vi "Periodic Tasks.vi"(8 "error in":errorcluster) -> ()   [LabVIEW 2014]
doc: "This VI runs in parallel to other tasks. It can contain as many user-defined periodic loops as you need. These can carry out PID or other sorts of timed response."
uses:
  <vilib>/Rock Robotics/WPI/DriverStation/WPI_DriverStationRobotMode2.ctl
  <vilib>/Rock Robotics/WPI/Joystick/WPI_JoystickGetSetRefNum.vi
  <vilib>/Rock Robotics/WPI/RobotDrive/WPI_RobotDriveGetSetRefNum.vi
  <vilib>/Rock Robotics/Network Tables/SD Read Number.vi
  Robot Global Data.vi
  <vilib>/Rock Robotics/Network Tables/SD Write Number.vi
  <vilib>/addons/control/pid/pid.llb/PID (DBL).vi
  <vilib>/Rock Robotics/WPI/Solenoid/Deprecated/WPI_SolenoidSetBool.vi
  <vilib>/Rock Robotics/WPI/RobotDrive/WPI_RobotDriveMecanumDrive_Cartesian.vi
  <vilib>/Rock Robotics/Network Tables/SD Write Numeric Array.vi
  <vilib>/Rock Robotics/Network Tables/SD Write Boolean Array.vi
  <vilib>/Rock Robotics/Network Tables/SD Write Boolean.vi
  <vilib>/addons/control/pid/NI_PID_pid.lvlib
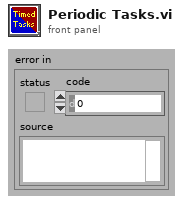
[diagram p1: front panel]
types:
  T1 = typedef "WPI_JoystickDevRef.ctl" = cluster{"Device":T2}
  T2 = typedef "WPI_JoystickDeviceEnum.ctl" = enum16{"USB 0", "USB 1", "USB 2", "USB 3", "USB 4", "USB 5"}
  T3 = typedef "WPI_RobotDriveDevRef.ctl" = cluster{"DevStatus":errorcluster, "Motors[]":T4[], "Square Inputs":bool, "Max Output":dbl}
  T4 = typedef "WPI_MotorControlDeviceRef.ctl" = cluster{"DeviceStatus":errorcluster, "Type":T5, "PWM":cluster{"Controller":T6, "PWM Channel":T7, "DeadBand":T8}, "CAN":cluster{"Device Number":u8, "Control Mode":T9, "Semaphore":T10, "Max Vout":dbl, "TalonSRX Control Mode":T11}, "Invert":bool, "TransformRef":T12, "InvTransformRef":T12}
  T5 = typedef "WPI_MotorControlType.ctl" = enum16{"PWM", "CAN", "CANTalonSRX"}
  T6 = typedef "FPGA_TypedefDigitalModule.ctl" = enum16{"Controller 1"}
  T7 = typedef "FPGA_DIOPWMChannel.ctl" = enum8{"PWM 0", "PWM 1", "PWM 2", "PWM 3", "PWM 4", "PWM 5", "PWM 6", "PWM 7", "PWM 8", "PWM 9", "PWM MXP 0", "PWM MXP 1", "PWM MXP 2", "PWM MXP 3", "PWM MXP 4", "PWM MXP 5", "PWM MXP 6", "PWM MXP 7", "PWM MXP 8", "PWM MXP 9", "Invalid"}
  T8 = typedef "WPI_PWMDeadband.ctl" = cluster{"Name":string, "maxPositivePwm":i32, "minPositivePwm":i32, "centerPwm":i32, "maxNegativePwm":i32, "minNegativePwm":i32, "angularRange":u16}
  T9 = typedef "WPI_CANJaguar_ControlMode.ctl" = enum8{"Percent VBus", "Current", "Speed", "Position", "Voltage"}
  T10 = typedef "Semaphore RefNum" = refnum<k1>
  T11 = typedef "WPI_CANTalonSRX_APIControlMode.ctl" = enum8{"Percent VBus", "Speed", "Position", "Slave", "Unchanged / Invalid"}
  T12 = typedef "WPI_PWMTransform_ConPane.ctl" = refnum<vi>
  T13 = typedef "WPI_EncoderDevRef.ctl" = cluster{"DevStatus":errorcluster, "EncoderIndex":T14, "CounterIndex":T15, "DistancePerCount":dbl, "Decoding Type":T16}
  T14 = typedef "FPGA_EncoderIdx.ctl" = enum8{"Enc 0", "Enc 1", "Enc 2", "Enc 3", "Enc 4", "Enc 5", "Enc 6", "Enc 7", "Invalid"}
  T15 = typedef "FPGA_CounterCtrSystemIndex.ctl" = enum8{"Ctr 0", "Ctr 1", "Ctr 2", "Ctr 3", "Ctr 4", "Ctr 5", "Ctr 6", "Ctr 7", "Invalid"}
  T16 = typedef "WPI_EncoderType.ctl" = enum16{"1x", "2x", "4x"}
  T17 = typedef "WPI_GyroDevRef.ctl" = cluster{"DevStatus":errorcluster, "Analog Module":T18, "Analog Channel":T19, "Offset":dbl, "Gain (VoltsPerDegree/Second)":dbl}
  T18 = typedef "FPGA_TypedefAnalogModule.ctl" = enum16{"Controller 1"}
  T19 = typedef "FPGA_AIChannel.ctl" = enum8{"AI 0", "AI 1", "AI 2", "AI 3", "AI MXP 0", "AI MXP 1", "AI MXP 2", "AI MXP 3", "Invalid"}
  T20 = typedef "WPI_SwitchDevRef.ctl" = cluster{"DevStatus":errorcluster, "DIO Channel":T21, "Controller":T6, "CntIndex":T15, "Normally Closed":bool}
  T21 = typedef "FPGA_DIOChannel.ctl" = enum8{"DIO 0", "DIO 1", "DIO 2", "DIO 3", "DIO 4", "DIO 5", "DIO 6", "DIO 7", "DIO 8", "DIO 9", "DIO MXP 0", "DIO MXP 1", "DIO MXP 2", "DIO MXP 3", "DIO MXP 4", "DIO MXP 5", "DIO MXP 6", "DIO MXP 7", "DIO MXP 8", "DIO MXP 9", "DIO MXP 10", "DIO MXP 11", "DIO MXP 12", "DIO MXP 13", "DIO MXP 14", "DIO MXP 15", "Invalid"}
  T22 = typedef "WPI_SolenoidDevRef.ctl" = cluster{"DevStatus":errorcluster, "Pneumatics Control Module":u8, "Forward Solenoid Channel":T23, "Reverse Solenoid Channel":T23}
  T23 = typedef "WPI_SolenoidChannel.ctl" = enum8{"Solenoid 0", "Solenoid 1", "Solenoid 2", "Solenoid 3", "Solenoid 4", "Solenoid 5", "Solenoid 6", "Solenoid 7", "Invalid"}
  T24 = cluster{"JoystickDevRef":T1, "RobotDriveDevRef":T3}
  T25 = cluster{"Buttons[0]":bool, "Buttons[1]":bool, "Buttons[2]":bool, "Buttons[3]":bool, "Buttons[4]":bool, "Buttons[5]":bool, "Buttons[6]":bool, "Buttons[7]":bool, "Buttons[8]":bool}
  T26 = typedef "WPI_DriverStationRobotMode2.ctl" = enum16{"Autonomous Disabled", "Autonomous Enabled", "Teleop Disabled", "Teleop Enabled", "Disconnected", "Finish", "Test Disabled", "Test Enabled", "Emergency Stopped"}
  T27 = cluster{"proportional gain (Kc)":dbl, "integral time (Ti, min)":dbl, "derivative time (Td, min)":dbl}
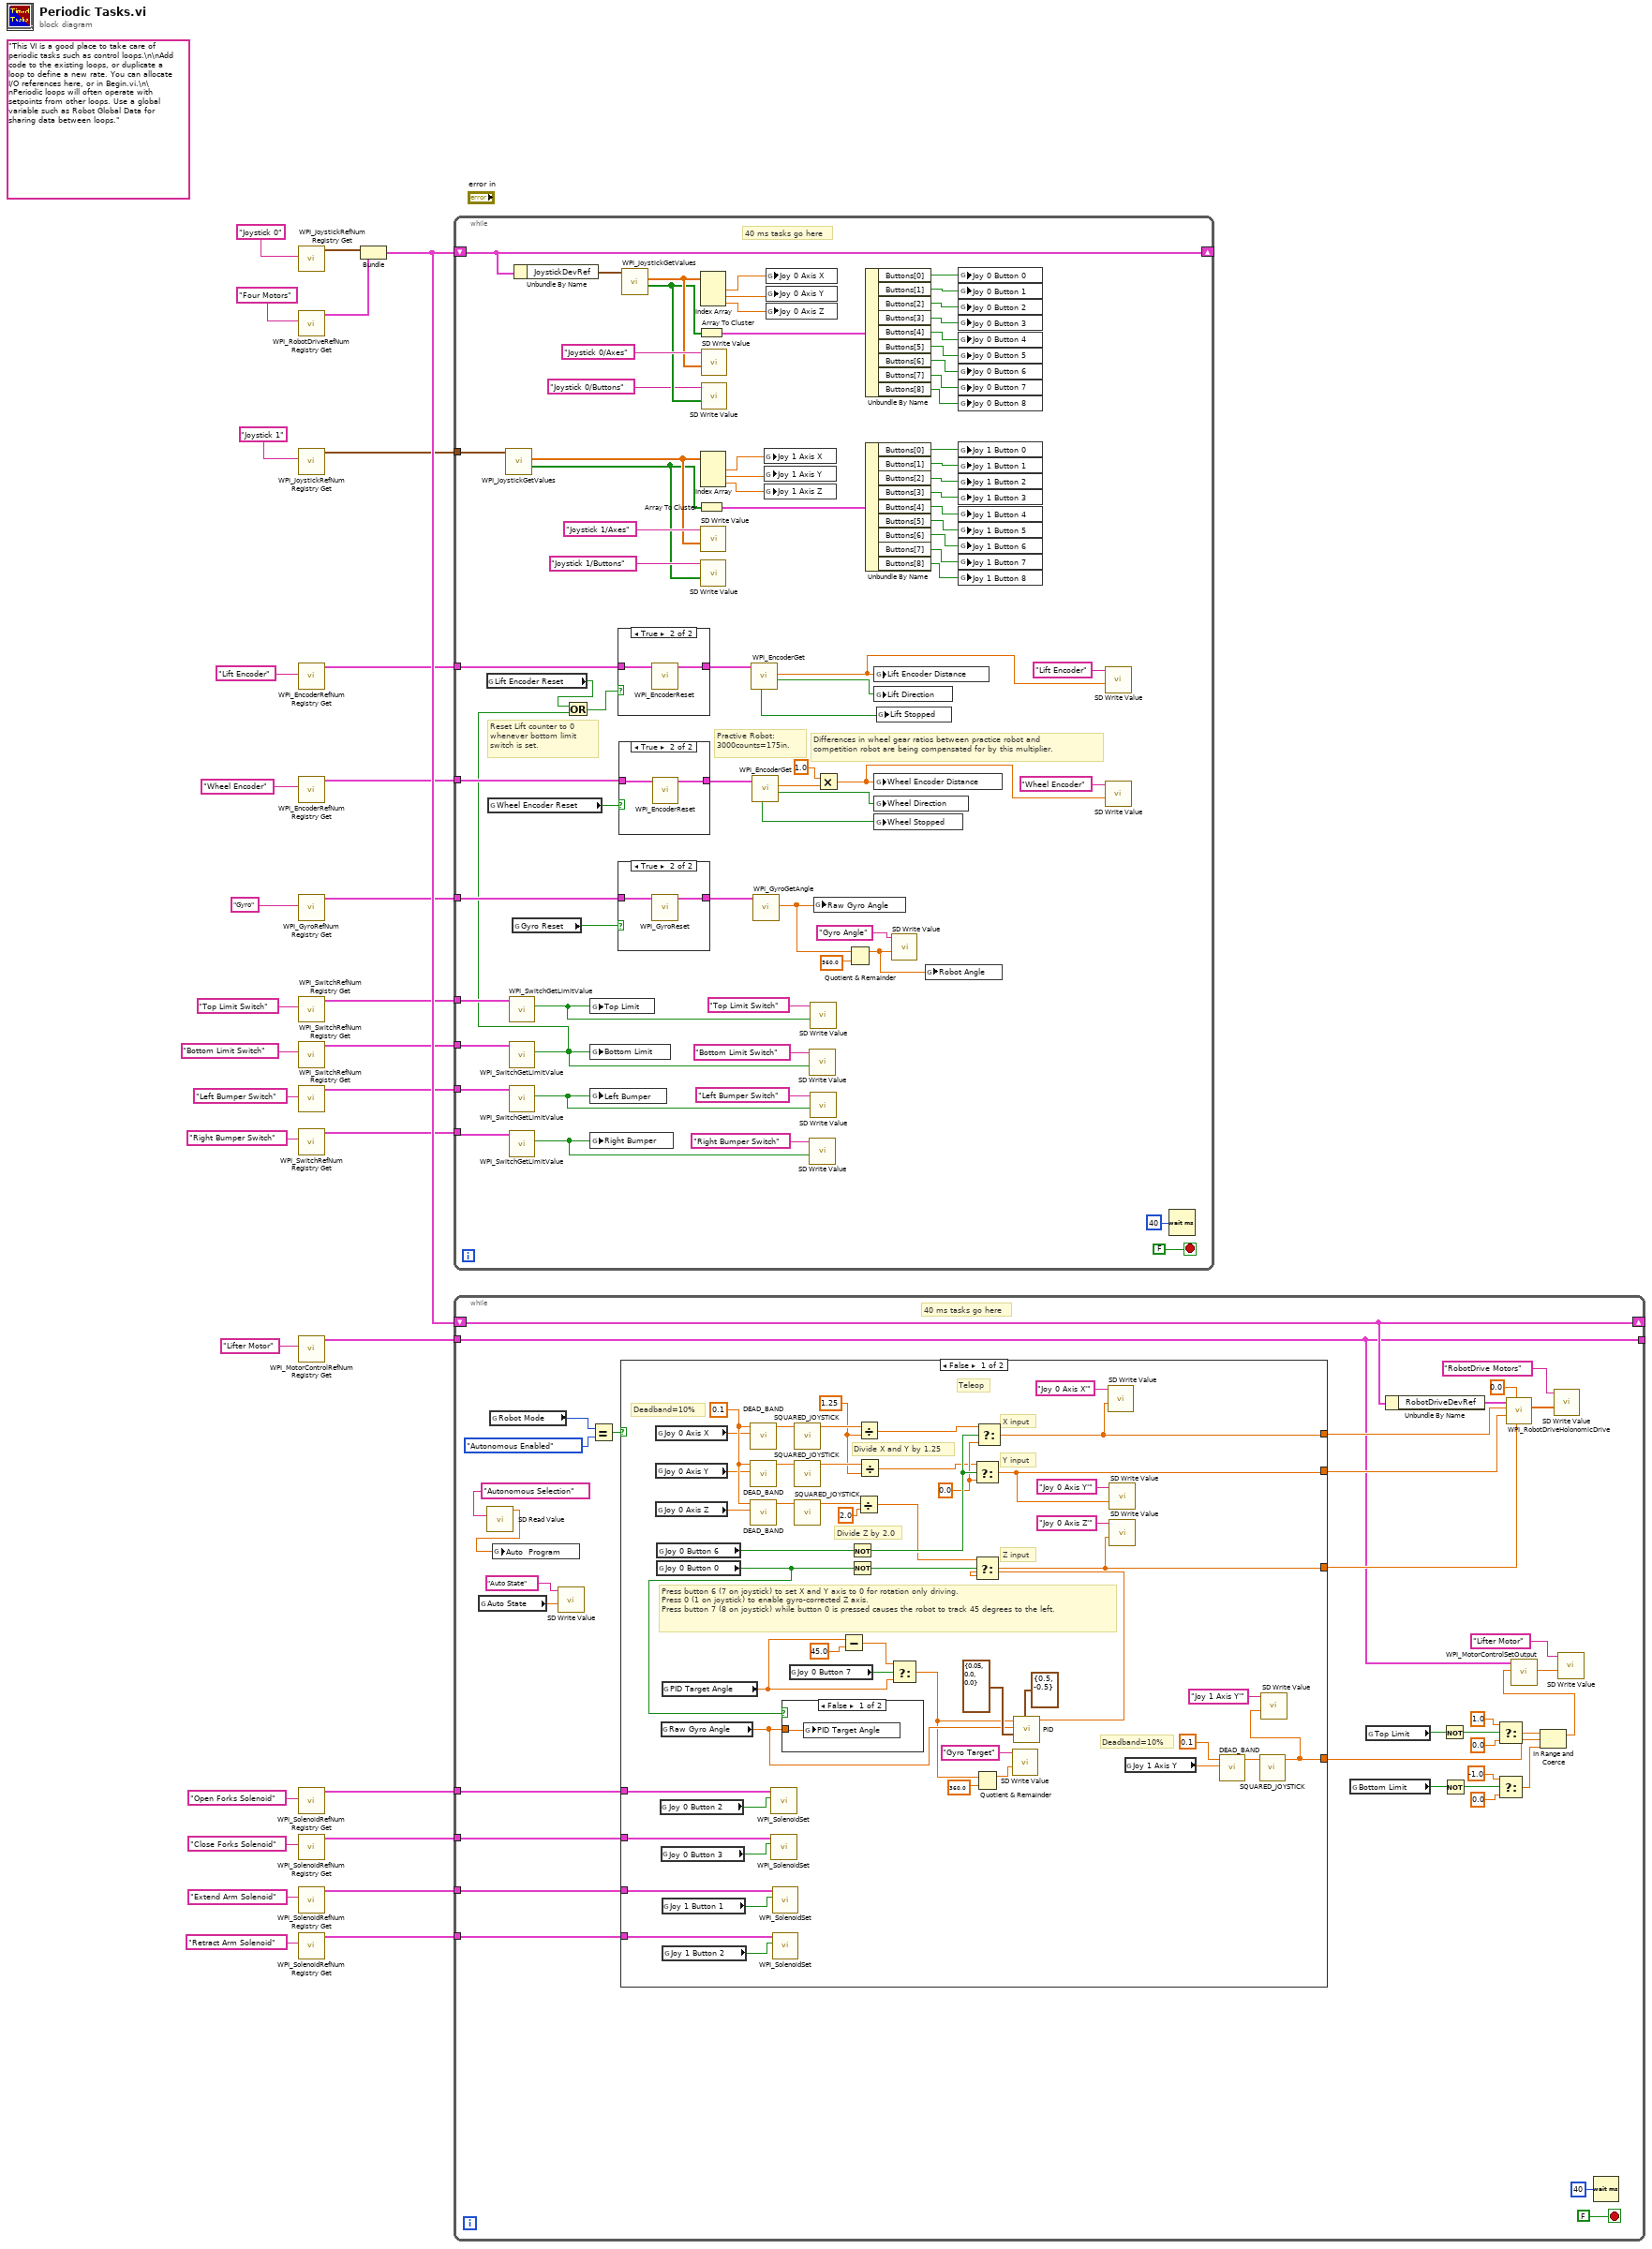
[diagram p0: block diagram]
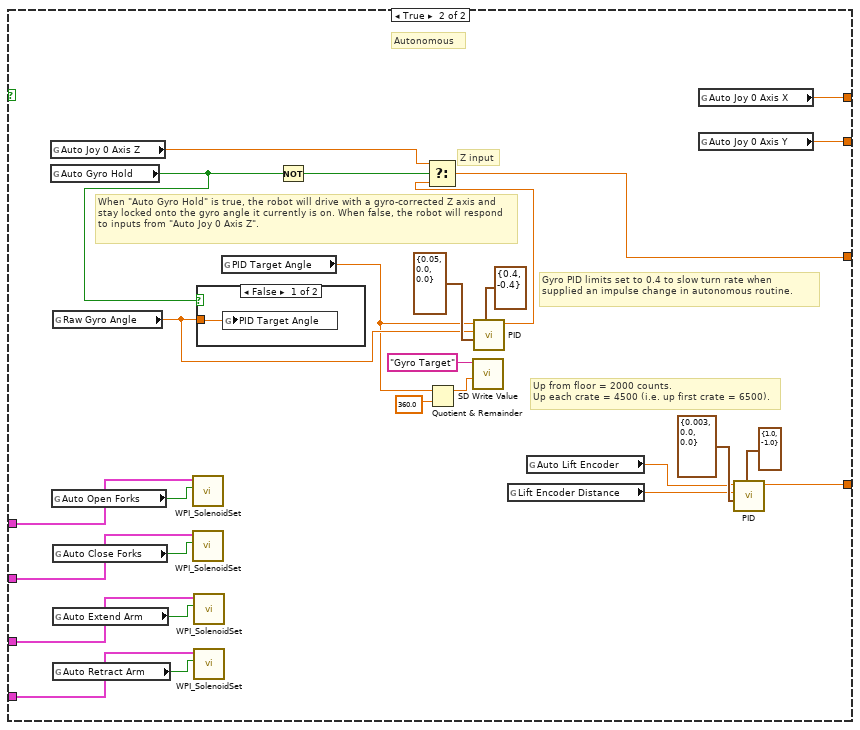
[diagram p3: hidden frame]
diagram:
  (unwired) "This VI is a good place to take care of periodic tasks such as control loops.\n\nAdd code to the existing loops, or duplicate a loop to define a new rate. You can allocate I/O references here, or in Begin.vi.\n\nPeriodic loops will often operate with setpoints from other loops. Use a global variable such as Robot Global Data for sharing data between loops."
  n1 = call <vilib>:"WPI_JoystickRefNum Registry Get.vi"("refnum name"="Joystick 0") -> ("JoystickDevRef"=w29:T1)  [unwired: 1 in, 9 out]
  n2 = call <vilib>:"WPI_RobotDriveRefNum Registry Get.vi"("refnum name"="Four Motors") -> ("RobotDriveDevRef"=w28:T3)  [unwired: 1 in, 9 out]
  n3 = call <vilib>:"WPI_JoystickRefNum Registry Get.vi"("refnum name"="Joystick 1") -> ("JoystickDevRef"=w25:T1)  [unwired: 1 in, 9 out]
  n4 = call <vilib>:"WPI_EncoderRefNum Registry Get.vi"("refnum name"="Lift Encoder") -> ("EncoderDevRef"=w21:T13)  [unwired: 9 in, 1 out]
  n5 = call <vilib>:"WPI_EncoderRefNum Registry Get.vi"("refnum name"="Wheel Encoder") -> ("EncoderDevRef"=w19:T13)  [unwired: 9 in, 1 out]
  n6 = call <vilib>:"WPI_GyroRefNum Registry Get.vi"("refnum name"="Gyro") -> ("GyroDevRef"=w23:T17)  [unwired: 9 in, 1 out]
  n7 = call <vilib>:"WPI_SwitchRefNum Registry Get.vi"("refnum name"="Top Limit Switch") -> ("SwitchDevRef"=w17:T20)  [unwired: 9 in, 1 out]
  n8 = call <vilib>:"WPI_SwitchRefNum Registry Get.vi"("refnum name"="Bottom Limit Switch") -> ("SwitchDevRef"=w16:T20)  [unwired: 9 in, 1 out]
  n9 = call <vilib>:"WPI_SwitchRefNum Registry Get.vi"("refnum name"="Left Bumper Switch") -> ("SwitchDevRef"=w2:T20)  [unwired: 9 in, 1 out]
  n10 = call <vilib>:"WPI_SwitchRefNum Registry Get.vi"("refnum name"="Right Bumper Switch") -> ("SwitchDevRef"=w1:T20)  [unwired: 9 in, 1 out]
  n11 = call <vilib>:"WPI_MotorControlRefNum Registry Get.vi"("refnum name"="Lifter Motor") -> ("MotorControlDevRef"=w5:T4)  [unwired: 9 in, 1 out]
  n12 = call <vilib>:"WPI_SolenoidRefNum Registry Get.vi"("refnum name"="Open Forks Solenoid") -> ("SolenoidDevRef"=w12:T22)  [unwired: 9 in, 1 out]
  n13 = call <vilib>:"WPI_SolenoidRefNum Registry Get.vi"("refnum name"="Close Forks Solenoid") -> ("SolenoidDevRef"=w11:T22)  [unwired: 9 in, 1 out]
  n14 = call <vilib>:"WPI_SolenoidRefNum Registry Get.vi"("refnum name"="Extend Arm Solenoid") -> ("SolenoidDevRef"=w8:T22)  [unwired: 9 in, 1 out]
  n15 = call <vilib>:"WPI_SolenoidRefNum Registry Get.vi"("refnum name"="Retract Arm Solenoid") -> ("SolenoidDevRef"=w7:T22)  [unwired: 9 in, 1 out]
  n16 = Bundle("JoystickDevRef"=w29, "RobotDriveDevRef"=w28) -> (w27:T24)  [unwired: 1 out]
  n17 = while {
    shift-right: [w104] -> _
    shift-left: w27 -> [w104]
    tunnel: w25 -> [w89]
    tunnel: w23 -> [w75]
    tunnel: w21 -> [w72]
    tunnel: w19 -> [w69]
    tunnel: w17 -> [w55]
    tunnel: w16 -> [w54]
    tunnel: w2 -> [w40]
    tunnel: w1 -> [w39]
    stop <- FALSE stop-if-true
    # "Practive Robot:\n3000counts=175in."
    # "Differences in wheel gear ratios between practice robot and competition robot are being compensated for by this multiplier."
    # "Reset Lift counter to 0 whenever bottom limit switch is set."
    # "40 ms tasks go here"
    n18 = global read "Robot Global Data.vi" "Lift Encoder Reset"() -> (w36:bool)
    n19 = global read "Robot Global Data.vi" "Wheel Encoder Reset"() -> (w70:bool)
    n20 = call <vilib>:"WPI_JoystickGetValues.vi"("JoystickDevRef"=w89) -> ("Buttons"=w60:bool[], "Axes"=w61:dbl[])  [unwired: 6 in, 3 out]
    n21 = call <vilib>:"WPI_SwitchGetLimitValue.vi"("SwitchDevRef"=w55) -> ("Switch Pressed"=w51:bool)  [unwired: 8 in, 2 out]
    n22 = call <vilib>:"WPI_SwitchGetLimitValue.vi"("SwitchDevRef"=w54) -> ("Switch Pressed"=w35:bool)  [unwired: 8 in, 2 out]
    n23 = call <vilib>:"WPI_SwitchGetLimitValue.vi"("SwitchDevRef"=w40) -> ("Switch Pressed"=w43:bool)  [unwired: 8 in, 2 out]
    n24 = call <vilib>:"WPI_SwitchGetLimitValue.vi"("SwitchDevRef"=w39) -> ("Switch Pressed"=w44:bool)  [unwired: 8 in, 2 out]
    n25 = global read "Robot Global Data.vi" "Gyro Reset"() -> (w73:bool)
    n26 = Unbundle By Name(w104) -> ("JoystickDevRef"=w103:T1)
    n27 = Or(x=w36, y=w35) -> (x .or. y?=w37:bool)
    n28 = global write "Robot Global Data.vi" "Top Limit"(w51) -> ()
    n29 = global write "Robot Global Data.vi" "Bottom Limit"(w35) -> ()
    n30 = global write "Robot Global Data.vi" "Left Bumper"(w43) -> ()
    n31 = global write "Robot Global Data.vi" "Right Bumper"(w44) -> ()
    n32 = case shown="True" w37 {
      tunnel: w72 -> [w110 w112]
      tunnel: [w110 w111] -> w71
      frame False {
      }
      frame True {
        n33 = call <vilib>:"WPI_EncoderReset.vi"("EncoderDevRef"=w112) -> ("EncoderDevRef"=w111:T13)  [unwired: 9 in, 1 out]
      }
    }
    n34 = case shown="True" w73 {
      tunnel: w75 -> [w113 w115]
      tunnel: [w113 w114] -> w74
      frame False {
      }
      frame True {
        n35 = call <vilib>:"WPI_GyroReset.vi"("GyroDevRef"=w115) -> ("GyroDevRef"=w114:T17)  [unwired: 9 in, 1 out]
      }
    }
    n36 = case shown="True" w70 {
      tunnel: w69 -> [w107 w108]
      tunnel: [w107 w109] -> w68
      frame False {
      }
      frame True {
        n37 = call <vilib>:"WPI_EncoderReset.vi"("EncoderDevRef"=w108) -> ("EncoderDevRef"=w109:T13)  [unwired: 9 in, 1 out]
      }
    }
    n38 = call <vilib>:"WPI_JoystickGetValues.vi"("JoystickDevRef"=w103) -> ("Buttons"=w65:bool[], "Axes"=w66:dbl[])  [unwired: 6 in, 3 out]
    n39 = Array To Cluster(array=w65) -> (cluster=w102:T25)
    n40 = Array To Cluster(array=w60) -> (cluster=w88:T25)
    n41 = Index Array(array=w66) -> (element #1=w92:dbl, element #2=w91:dbl, element #3=w90:dbl)  [unwired: 3 in]
    n42 = Index Array(array=w61) -> (element #1=w78:dbl, element #2=w77:dbl, element #3=w76:dbl)  [unwired: 3 in]
    n43 = call-poly <vilib>:"SD Write Value.vi"("Numeric Array"=w61, "Name"="Joystick 1/Axes") -> ()  [unwired: 8 in, 2 out]
    n44 = call-poly <vilib>:"SD Write Value.vi"("Boolean Array"=w60, "Name"="Joystick 1/Buttons") -> ()  [unwired: 8 in, 2 out]
    n45 = call-poly <vilib>:"SD Write Value.vi"("Numeric Array"=w66, "Name"="Joystick 0/Axes") -> ()  [unwired: 8 in, 2 out]
    n46 = call-poly <vilib>:"SD Write Value.vi"("Boolean Array"=w65, "Name"="Joystick 0/Buttons") -> ()  [unwired: 8 in, 2 out]
    n47 = call <vilib>:"WPI_EncoderGet.vi"("EncoderDevRef"=w71) -> ("Direction"=w50:bool, "Distance"=w38:dbl, "Stopped"=w49:bool)  [unwired: 5 in, 3 out]
    n48 = call <vilib>:"WPI_EncoderGet.vi"("EncoderDevRef"=w68) -> ("Direction"=w48:bool, "Distance"=w34:dbl, "Stopped"=w47:bool)  [unwired: 5 in, 3 out]
    n49 = call <vilib>:"WPI_GyroGetAngle.vi"("GyroDevRef"=w74) -> ("Angle"=w57:dbl)  [unwired: 7 in, 3 out]
    n50 = global write "Robot Global Data.vi" "Joy 1 Axis X"(w78) -> ()
    n51 = global write "Robot Global Data.vi" "Joy 1 Axis Y"(w77) -> ()
    n52 = global write "Robot Global Data.vi" "Joy 1 Axis Z"(w76) -> ()
    n53 = global write "Robot Global Data.vi" "Joy 0 Axis X"(w92) -> ()
    n54 = global write "Robot Global Data.vi" "Joy 0 Axis Y"(w91) -> ()
    n55 = global write "Robot Global Data.vi" "Joy 0 Axis Z"(w90) -> ()
    n56 = call-poly <vilib>:"SD Write Value.vi"("Boolean"=w35, "Name"="Bottom Limit Switch") -> ()  [unwired: 8 in, 2 out]
    n57 = call-poly <vilib>:"SD Write Value.vi"("Boolean"=w44, "Name"="Right Bumper Switch") -> ()  [unwired: 8 in, 2 out]
    n58 = call-poly <vilib>:"SD Write Value.vi"("Boolean"=w51, "Name"="Top Limit Switch") -> ()  [unwired: 8 in, 2 out]
    n59 = call-poly <vilib>:"SD Write Value.vi"("Boolean"=w43, "Name"="Left Bumper Switch") -> ()  [unwired: 8 in, 2 out]
    n60 = global write "Robot Global Data.vi" "Raw Gyro Angle"(w57) -> ()
    n61 = Multiply(x=1.0, y=w34) -> (x*y=w33:dbl)
    n62 = Quotient & Remainder(x=w57, y=360.0) -> (x-y*floor(x/y)=w56:dbl)  [unwired: 1 out]
    n63 = Unbundle By Name(w102) -> ("Buttons[0]"=w101:bool, "Buttons[1]"=w100:bool, "Buttons[2]"=w99:bool, "Buttons[3]"=w98:bool, "Buttons[4]"=w97:bool, "Buttons[5]"=w96:bool, "Buttons[6]"=w95:bool, "Buttons[7]"=w94:bool, "Buttons[8]"=w93:bool)
    n64 = Unbundle By Name(w88) -> ("Buttons[0]"=w87:bool, "Buttons[1]"=w86:bool, "Buttons[2]"=w85:bool, "Buttons[3]"=w84:bool, "Buttons[4]"=w83:bool, "Buttons[5]"=w82:bool, "Buttons[6]"=w81:bool, "Buttons[7]"=w80:bool, "Buttons[8]"=w79:bool)
    n65 = global write "Robot Global Data.vi" "Lift Encoder Distance"(w38) -> ()
    n66 = global write "Robot Global Data.vi" "Lift Direction"(w50) -> ()
    n67 = global write "Robot Global Data.vi" "Wheel Encoder Distance"(w33) -> ()
    n68 = global write "Robot Global Data.vi" "Wheel Direction"(w48) -> ()
    n69 = global write "Robot Global Data.vi" "Wheel Stopped"(w47) -> ()
    n70 = global write "Robot Global Data.vi" "Lift Stopped"(w49) -> ()
    n71 = call-poly <vilib>:"SD Write Value.vi"("Numeric"=w56, "Name"="Gyro Angle") -> ()  [unwired: 8 in, 2 out]
    n72 = global write "Robot Global Data.vi" "Robot Angle"(w56) -> ()
    n73 = global write "Robot Global Data.vi" "Joy 0 Button 0"(w101) -> ()
    n74 = global write "Robot Global Data.vi" "Joy 0 Button 1"(w100) -> ()
    n75 = global write "Robot Global Data.vi" "Joy 0 Button 2"(w99) -> ()
    n76 = global write "Robot Global Data.vi" "Joy 0 Button 3"(w98) -> ()
    n77 = global write "Robot Global Data.vi" "Joy 0 Button 4"(w97) -> ()
    n78 = global write "Robot Global Data.vi" "Joy 0 Button 5"(w96) -> ()
    n79 = global write "Robot Global Data.vi" "Joy 0 Button 6"(w95) -> ()
    n80 = global write "Robot Global Data.vi" "Joy 0 Button 7"(w94) -> ()
    n81 = global write "Robot Global Data.vi" "Joy 0 Button 8"(w93) -> ()
    n82 = global write "Robot Global Data.vi" "Joy 1 Button 0"(w87) -> ()
    n83 = global write "Robot Global Data.vi" "Joy 1 Button 1"(w86) -> ()
    n84 = global write "Robot Global Data.vi" "Joy 1 Button 2"(w85) -> ()
    n85 = global write "Robot Global Data.vi" "Joy 1 Button 3"(w84) -> ()
    n86 = global write "Robot Global Data.vi" "Joy 1 Button 4"(w83) -> ()
    n87 = global write "Robot Global Data.vi" "Joy 1 Button 5"(w82) -> ()
    n88 = global write "Robot Global Data.vi" "Joy 1 Button 6"(w81) -> ()
    n89 = global write "Robot Global Data.vi" "Joy 1 Button 7"(w80) -> ()
    n90 = global write "Robot Global Data.vi" "Joy 1 Button 8"(w79) -> ()
    n91 = call-poly <vilib>:"SD Write Value.vi"("Numeric"=w38, "Name"="Lift Encoder") -> ()  [unwired: 8 in, 2 out]
    n92 = call-poly <vilib>:"SD Write Value.vi"("Numeric"=w33, "Name"="Wheel Encoder") -> ()  [unwired: 8 in, 2 out]
    n93 = Wait (ms)(milliseconds to wait=u32 40) -> ()  [unwired: 1 out]
  }
  n94 = while {
    shift-right: [w146] -> _
    shift-left: w27 -> [w146]
    tunnel: w12 -> [w138]
    tunnel: w11 -> [w137]
    tunnel: w8 -> [w136]
    tunnel: w7 -> [w135]
    tunnel: [w134] -> _
    tunnel: w5 -> [w134]
    stop <- FALSE stop-if-true
    # "40 ms tasks go here"
    n95 = global read "Robot Global Data.vi" "Auto State"() -> (w117:dbl)
    n96 = call-poly <vilib>:"SD Read Value.vi"("Name"="Autonomous Selection") -> ("Numeric"=w118:dbl)  [unwired: 8 in, 2 out]
    n97 = global read "Robot Global Data.vi" "Robot Mode"() -> (w140:T26)
    n98 = global write "Robot Global Data.vi" "Auto  Program"(w118) -> ()
    n99 = call-poly <vilib>:"SD Write Value.vi"("Numeric"=w117, "Name"="Auto State") -> ()  [unwired: 8 in, 2 out]
    n100 = Equal?(x=w140, y=WPI_DriverStationRobotMode2."Autonomous Enabled") -> (x = y?=w141:bool)
    n101 = case shown="False" w141 {
      tunnel: [w191 w230] -> w144
      tunnel: [w188 w229] -> w143
      tunnel: [w187 w208] -> w142
      tunnel: w138 -> [w179 w228]
      tunnel: w137 -> [w178 w227]
      tunnel: w136 -> [w175 w222]
      tunnel: w135 -> [w174 w221]
      tunnel: [w163 w218] -> w120
      frame False {
        w157 = 1.25 ("y")
        w199 = 0.1 ("deadband input")
        w201 = 0.0
        # "Divide X and Y by 1.25"
        # "Deadband=10%"
        # "Deadband=10%"
        # "Divide Z by 2.0"
        # "Z input"
        # "Y input"
        # "X input"
        # "Press button 6 (7 on joystick) to set X and Y axis to 0 for rotation only driving.\nPress 0 (1 on joystick) to enable gyro-corrected Z axis.\nPress button 7 (8 on joystick) while button 0 is pressed causes the robot to track 45 degrees to the left."
        # "Teleop"
        n102 = global read "Robot Global Data.vi" "Joy 0 Axis X"() -> (w196:dbl)
        n103 = global read "Robot Global Data.vi" "Joy 0 Axis Y"() -> (w195:dbl)
        n104 = global read "Robot Global Data.vi" "Joy 0 Axis Z"() -> (w194:dbl)
        n105 = global read "Robot Global Data.vi" "Joy 0 Button 6"() -> (w193:bool)
        n106 = global read "Robot Global Data.vi" "Joy 0 Button 0"() -> (w183:bool)
        n107 = global read "Robot Global Data.vi" "Joy 0 Button 2"() -> (w181:bool)
        n108 = global read "Robot Global Data.vi" "Raw Gyro Angle"() -> (w182:dbl)
        n109 = global read "Robot Global Data.vi" "Joy 0 Button 3"() -> (w180:bool)
        n110 = global read "Robot Global Data.vi" "PID Target Angle"() -> (w153:dbl)
        n111 = global read "Robot Global Data.vi" "Joy 1 Button 1"() -> (w177:bool)
        n112 = global read "Robot Global Data.vi" "Joy 1 Button 2"() -> (w176:bool)
        n113 = call "DEAD_BAND.vi"("axis input"=w196, "deadband input"=w199) -> ("axis output"=w167:dbl)  [unwired: 9 in]
        n114 = call "DEAD_BAND.vi"("axis input"=w195, "deadband input"=w199) -> ("axis output"=w166:dbl)  [unwired: 9 in]
        n115 = call "DEAD_BAND.vi"("axis input"=w194, "deadband input"=w199) -> ("axis output"=w165:dbl)  [unwired: 9 in]
        n116 = call-poly <vilib>:"WPI_SolenoidSet.vi"("Value"=w181, "SolenoidDevRef"=w179) -> ()  [unwired: 8 in, 2 out]
        n117 = call-poly <vilib>:"WPI_SolenoidSet.vi"("Value"=w180, "SolenoidDevRef"=w178) -> ()  [unwired: 8 in, 2 out]
        n118 = call-poly <vilib>:"WPI_SolenoidSet.vi"("Value"=w177, "SolenoidDevRef"=w175) -> ()  [unwired: 8 in, 2 out]
        n119 = call-poly <vilib>:"WPI_SolenoidSet.vi"("Value"=w176, "SolenoidDevRef"=w174) -> ()  [unwired: 8 in, 2 out]
        n120 = case shown="False" w183 {
          tunnel: w182 -> [w203 _]
          frame False {
            n121 = global write "Robot Global Data.vi" "PID Target Angle"(w203) -> ()
          }
          frame True {
          }
        }
        n122 = global read "Robot Global Data.vi" "Joy 0 Button 7"() -> (w155:bool)
        n123 = call "SQUARED_JOYSTICK.vi"("axis input"=w167) -> ("axis output"=w161:dbl)  [unwired: 10 in]
        n124 = call "SQUARED_JOYSTICK.vi"("axis input"=w166) -> ("axis output"=w159:dbl)  [unwired: 10 in]
        n125 = call "SQUARED_JOYSTICK.vi"("axis input"=w165) -> ("axis output"=w164:dbl)  [unwired: 10 in]
        n126 = Subtract(x=w153, y=45.0) -> (x-y=w152:dbl)
        n127 = Not(x=w193) -> (.not. x?=w202:bool)
        n128 = Not(x=w183) -> (.not. x?=w200:bool)
        n129 = Divide(x=w164, y=2.0) -> (x/y=w197:dbl)
        n130 = Divide(x=w161, y=w157) -> (x/y=w160:dbl)
        n131 = Divide(x=w159, y=w157) -> (x/y=w158:dbl)
        n132 = Select(t=w152, s=w155, f=w153) -> (s? t:f=w156:dbl)
        n133 = Select(t=w158, s=w202, f=w201) -> (s? t:f=w188:dbl)
        n134 = Quotient & Remainder(x=w156, y=360.0) -> (x-y*floor(x/y)=w168:dbl)  [unwired: 1 out]
        n135 = Select(t=w160, s=w202, f=w201) -> (s? t:f=w191:dbl)
        n136 = call-poly <vilib>:"SD Write Value.vi"("Numeric"=w168, "Name"="Gyro Target") -> ()  [unwired: 8 in, 2 out]
        n137 = call-poly <vilib>:"PID.vi"("output range"=cluster{"output high":dbl, "output low":dbl} {"output high"=0.5, "output low"=-0.5}, "PID gains"=T27 {"proportional gain (Kc)"=0.05, "integral time (Ti, min)"=0.0, "derivative time (Td, min)"=0.0}, "process variable"=w182, "setpoint"=w156) -> ("output"=w184:dbl)  [unwired: 6 in, 1 out]
        n138 = Select(t=w197, s=w200, f=w184) -> (s? t:f=w187:dbl)
        n139 = call-poly <vilib>:"SD Write Value.vi"("Numeric"=w191, "Name"="Joy 0 Axis X'") -> ()  [unwired: 8 in, 2 out]
        n140 = call-poly <vilib>:"SD Write Value.vi"("Numeric"=w188, "Name"="Joy 0 Axis Y'") -> ()  [unwired: 8 in, 2 out]
        n141 = call-poly <vilib>:"SD Write Value.vi"("Numeric"=w187, "Name"="Joy 0 Axis Z'") -> ()  [unwired: 8 in, 2 out]
        n142 = global read "Robot Global Data.vi" "Joy 1 Axis Y"() -> (w172:dbl)
        n143 = call "DEAD_BAND.vi"("axis input"=w172, "deadband input"=0.1) -> ("axis output"=w162:dbl)  [unwired: 9 in]
        n144 = call "SQUARED_JOYSTICK.vi"("axis input"=w162) -> ("axis output"=w163:dbl)  [unwired: 10 in]
        n145 = call-poly <vilib>:"SD Write Value.vi"("Numeric"=w163, "Name"="Joy 1 Axis Y'") -> ()  [unwired: 8 in, 2 out]
      }
      frame True {
        # "Gyro PID limits set to 0.4 to slow turn rate when \nsupplied an impulse change in autonomous routine."
        # "Z input"
        # "When \"Auto Gyro Hold\" is true, the robot will drive with a gyro-corrected Z axis and stay locked onto the gyro angle it currently is on. When false, the robot will respond to inputs from \"Auto Joy 0 Axis Z\"."
        # "Up from floor = 2000 counts.\nUp each crate = 4500 (i.e. up first crate = 6500)."
        # "Autonomous"
        n146 = global read "Robot Global Data.vi" "Auto Joy 0 Axis Z"() -> (w209:dbl)
        n147 = global read "Robot Global Data.vi" "Auto Gyro Hold"() -> (w211:bool)
        n148 = global read "Robot Global Data.vi" "Auto Open Forks"() -> (w226:bool)
        n149 = global read "Robot Global Data.vi" "Raw Gyro Angle"() -> (w210:dbl)
        n150 = global read "Robot Global Data.vi" "Auto Close Forks"() -> (w225:bool)
        n151 = global read "Robot Global Data.vi" "Auto Extend Arm"() -> (w224:bool)
        n152 = global read "Robot Global Data.vi" "Auto Retract Arm"() -> (w223:bool)
        n153 = call-poly <vilib>:"WPI_SolenoidSet.vi"("Value"=w226, "SolenoidDevRef"=w228) -> ()  [unwired: 8 in, 2 out]
        n154 = call-poly <vilib>:"WPI_SolenoidSet.vi"("Value"=w225, "SolenoidDevRef"=w227) -> ()  [unwired: 8 in, 2 out]
        n155 = call-poly <vilib>:"WPI_SolenoidSet.vi"("Value"=w224, "SolenoidDevRef"=w222) -> ()  [unwired: 8 in, 2 out]
        n156 = call-poly <vilib>:"WPI_SolenoidSet.vi"("Value"=w223, "SolenoidDevRef"=w221) -> ()  [unwired: 8 in, 2 out]
        n157 = case shown="False" w211 {
          tunnel: w210 -> [w231 _]
          frame False {
            n158 = global write "Robot Global Data.vi" "PID Target Angle"(w231) -> ()
          }
          frame True {
          }
        }
        n159 = global read "Robot Global Data.vi" "PID Target Angle"() -> (w204:dbl)
        n160 = Not(x=w211) -> (.not. x?=w215:bool)
        n161 = Quotient & Remainder(x=w204, y=360.0) -> (x-y*floor(x/y)=w205:dbl)  [unwired: 1 out]
        n162 = call-poly <vilib>:"SD Write Value.vi"("Numeric"=w205, "Name"="Gyro Target") -> ()  [unwired: 8 in, 2 out]
        n163 = call-poly <vilib>:"PID.vi"("output range"=cluster{"output high":dbl, "output low":dbl} {"output high"=0.4, "output low"=-0.4}, "PID gains"=T27 {"proportional gain (Kc)"=0.05, "integral time (Ti, min)"=0.0, "derivative time (Td, min)"=0.0}, "process variable"=w210, "setpoint"=w204) -> ("output"=w212:dbl)  [unwired: 6 in, 1 out]
        n164 = Select(t=w209, s=w215, f=w212) -> (s? t:f=w208:dbl)
        n165 = global read "Robot Global Data.vi" "Lift Encoder Distance"() -> (w217:dbl)
        n166 = global read "Robot Global Data.vi" "Auto Lift Encoder"() -> (w216:dbl)
        n167 = global read "Robot Global Data.vi" "Auto Joy 0 Axis X"() -> (w230:dbl)
        n168 = global read "Robot Global Data.vi" "Auto Joy 0 Axis Y"() -> (w229:dbl)
        n169 = call-poly <vilib>:"PID.vi"("output range"=cluster{"output high":dbl, "output low":dbl} {"output high"=1.0, "output low"=-1.0}, "PID gains"=T27 {"proportional gain (Kc)"=0.003, "integral time (Ti, min)"=0.0, "derivative time (Td, min)"=0.0}, "process variable"=w217, "setpoint"=w216) -> ("output"=w218:dbl)  [unwired: 6 in, 1 out]
      }
    }
    n170 = global read "Robot Global Data.vi" "Bottom Limit"() -> (w131:bool)
    n171 = global read "Robot Global Data.vi" "Top Limit"() -> (w130:bool)
    n172 = Unbundle By Name(w146) -> ("RobotDriveDevRef"=w145:T3)
    n173 = Not(x=w130) -> (.not. x?=w128:bool)
    n174 = Not(x=w131) -> (.not. x?=w129:bool)
    n175 = Select(t=1.0, s=w128, f=0.0 ("t")) -> (s? t:f=w126:dbl)
    n176 = Select(t=-1.0, s=w129, f=0.0 ("t")) -> (s? t:f=w127:dbl)
    n177 = call-poly <vilib>:"WPI_RobotDriveHolonomicDrive.vi"("Rotation"=w142, "Gyro Angle"=0.0, "Y"=w143, "X"=w144, "RobotDriveDevRef"=w145) -> ("Motor Values"=w148:dbl[])  [unwired: 4 in, 2 out]
    n178 = In Range and Coerce(upper limit=w126, x=w120, lower limit=w127) -> (coerced(x)=w121:dbl)  [unwired: 1 out]
    n179 = call <vilib>:"WPI_MotorControlSetOutput.vi"("Output"=w121, "MotorControlDevRef"=w134) -> ("Motor Output"=w133:dbl)  [unwired: 7 in, 2 out]
    n180 = call-poly <vilib>:"SD Write Value.vi"("Numeric Array"=w148, "Name"="RobotDrive Motors") -> ()  [unwired: 8 in, 2 out]
    n181 = call-poly <vilib>:"SD Write Value.vi"("Numeric"=w133, "Name"="Lifter Motor") -> ()  [unwired: 8 in, 2 out]
    n182 = Wait (ms)(milliseconds to wait=u32 40) -> ()  [unwired: 1 out]
  }
